vi "TagStringValuesUpdatedBroadcast_Parse.vi"(8 "error in (no error)":errorcluster, 11 "Message":T7) -> (0 "error out":errorcluster, 1 "Body":T1, 2 "Header":T5, 3 "TagStringValuesUpdatedBroadcast":T4)   [LabVIEW 2017]
uses:
  <vilib>/addons/InsightCM/MessageBus/Base/controls/Message.ctl
  <vilib>/addons/InsightCM/MessageBus/Base/controls/MessageHeader.ctl
  <vilib>/addons/InsightCM/MessageBus/Base/controls/KeyValuePair.ctl
  <vilib>/addons/InsightCM/MessageBus/MessageLibrary/Tag/controls/TagStringValuesUpdatedBroadcast.ctl
  <vilib>/addons/InsightCM/MessageBus/MessageLibrary/Tag/controls/TagStringValuesUpdatedBroadcastBody.ctl
  <vilib>/addons/InsightCM/MessageBus/Base/controls/TagValueString.ctl
  <vilib>/addons/InsightCM/MessageBus/Base/controls/TsTagValueString.ctl
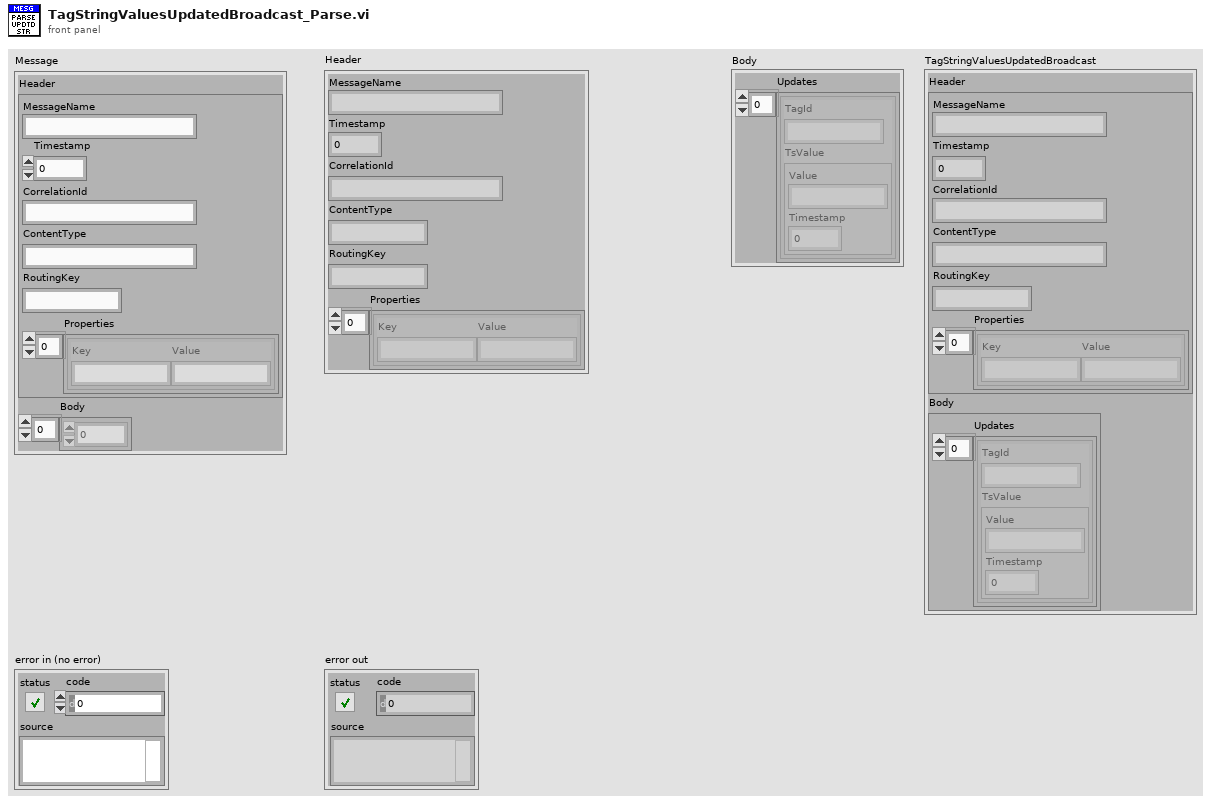
[diagram p1: front panel]
types:
  T1 = typedef "TagStringValuesUpdatedBroadcastBody.ctl" = cluster{"Updates":T2[]}
  T2 = typedef "TagValueString.ctl" = cluster{"TagId":string, "TsValue":T3}
  T3 = typedef "TsTagValueString.ctl" = cluster{"Value":string, "Timestamp":i64}
  T4 = typedef "TagStringValuesUpdatedBroadcast.ctl" = cluster{"Header":T5, "Body":T1}
  T5 = typedef "MessageHeader.ctl" = cluster{"MessageName":string, "Timestamp":i64, "CorrelationId":string, "ContentType":string, "RoutingKey":string, "Properties":T6[]}
  T6 = typedef "KeyValuePair.ctl" = cluster{"Key":string, "Value":string}
  T7 = typedef "Message.ctl" = cluster{"Header":T5, "Body":u8[]}
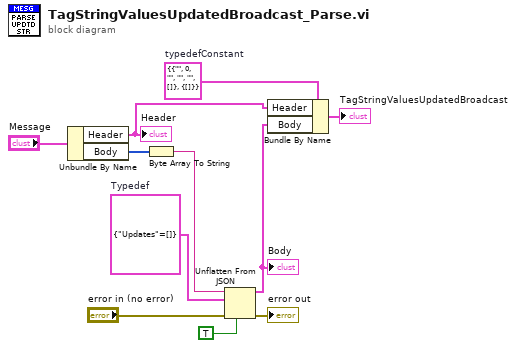
[diagram p0: block diagram]
diagram:
  w3 = T4 {"Header"={"MessageName"="", "Timestamp"=0, "CorrelationId"="", "ContentType"="", "RoutingKey"="", "Properties"=[]}, "Body"={"Updates"=[]}}  # typedefConstant
  w7 = T1 {"Updates"=[]}  # Typedef
  n1 = Unbundle By Name("Message") -> ("Header"=w9:T5, "Body"=w1:u8[])
  "Header" <- w9
  n2 = Byte Array To String(unsigned byte array=w1) -> (string=w6:string)
  n3 = Unflatten From JSON(JSON string=w6, type and defaults=w7, default null elements? (F)=TRUE, error in (no error)="error in (no error)") -> (value=w5:T1, error out=→"error out":errorcluster)  [unwired: 3 in]
  "Body" <- w5
  n4 = Bundle By Name(cluster=w3, "Header"=w9, "Body"=w5) -> (→"TagStringValuesUpdatedBroadcast":T4)
